vi "Set Datatype group.vi"(8 "error in (no error)":errorcluster, 10 "Datatype group in":refnum<class "Datatype group.lvclass">, 11 "Channel group in":refnum<class "Channel group.lvclass">) -> (0 "error out":errorcluster, 2 "replaced":bool, 3 "Channel group out":refnum<class "Channel group.lvclass">)   [LabVIEW 2016, in "FPGA RM Shared API.lvlib" / "Channel group.lvclass"]
uses:
  Channel group.lvclass
  Datatype Group/Datatype group.lvclass
  Datatype Group/Datatype group.lvclass/Datatype group.ctl
  Channel group.lvclass/Channel group.ctl
  Datatype Group/Read datatype.vi
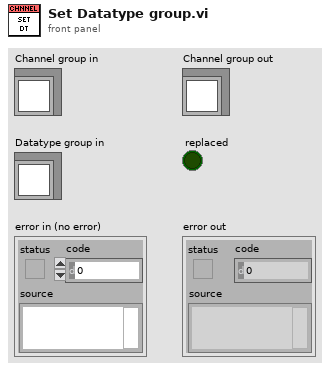
[diagram p1: front panel]
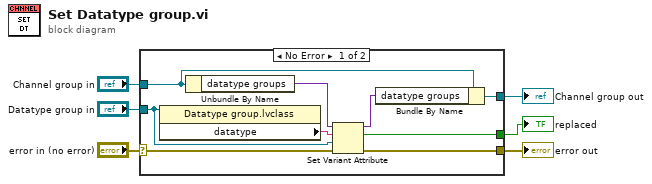
[diagram p0: block diagram]
diagram:
  n1 = case shown="No Error" "error in (no error)" {
    selector: "error in (no error)" -> [w11 w17]
    tunnel: [w10 w17] -> w5
    tunnel: [w14 w16] -> w3
    tunnel: "Channel group in" -> [w15 w16]
    tunnel: "Datatype group in" -> [w8 _]
    tunnel: [w9 _] -> w1
    frame No Error {
      n2 = property class="Datatype group.lvclass"(reference=w8) -> ("datatype"=w7:string)  [unwired: 1 in, 2 out]
      n3 = Unbundle By Name(w15) -> ("datatype groups"=w13:variant)
      n4 = Set Variant Attribute(Variant=w13, name=w7, value=w8, error in=w11) -> (Variant out=w12:variant, replaced=w9:bool, error out=w10:errorcluster)
      n5 = Bundle By Name(cluster=w15, "datatype groups"=w12) -> (w14:refnum<class "Channel group.lvclass">)
    }
    frame Error {
    }
  }
  "error out" <- w5
  "Channel group out" <- w3
  "replaced" <- w1
